vi "GSI-HVSwitch2.set high voltage.vi"(0 "i ref in":refnum<vi>, 2 "High Voltage":dbl format="%.2f", 3 "ms timeout (10000)":i32=10000, 5 "error in (no error)":errorcluster) -> (14 "i ref out":refnum<vi>, 17 "timed out":bool, 19 "error out":errorcluster)   [LabVIEW 2014, in "GSI-HVSwitch2.lvlib"]
doc: "Sets the voltage value for the logic \"High\" state."
uses:
  GSI-HVSwitch2.lvlib
  CSCore/CSSystem/CoreDefs/CoreDefs.error_type.ctl
  CSCore/CSSystem/CoreDefs/CoreDefs.error_severity.ctl
  CSlibraries-extern/DimLVEvent/LVDimInterface/LVDimInterface.lvlib
  CSCore/CSSystem/CoreLib/CoreLib.lvlib
  CSlibraries/UtilityLib/UtilityLib.lvlib
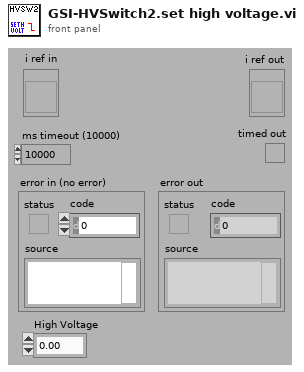
[diagram p1: front panel]
types:
  T1 = typedef "CoreDefs.error_severity.ctl" = enum16{"undefined", "information", "warning", "error", "fatal"}
  T2 = typedef "CoreDefs.error_type.ctl" = enum16{"no error", "can't load process", "can't unload process", "process does not exist", "can't install process", "can't remove process", "unknown function", "time out", "can't execute function", "duplicate queue name", "super not found", "caller queue invalid", "can't ping process", "unknown error", "VISA Error", "VISA timeout", "GPIB timeout", "GPIB error", "communication error", "data type mismatch", "can't read data from OPC server", "can't write data to OPC server", "OET error", "function not implemented", "process already exists", "invalid Shared Variable name", "error writing Shared Variable", "error reading Shared Variable", "invalid client name", "corrupt database", "unknown class", "call not authorized", "parameter out of range", "OET timeout: can't get data to modify", "invalid queue name", "requested operation incompatible with current state", "event undefined", "event disabled", "state undefined", "caller is not a friend", "EventBuilder: bad eventID", "EventBuilder: no DAQ devices", "a thread must not stop itself", "UNUSED ELEMENT4", "DiscArchiver: eventData incomplete", "DiscArchiver: eventData does not belong to run", "DiscArchiver: can't open file", "DiscArchiver: can't write to file", "DiscArchiver: available disc space low", "can't acquire semaphore", "error reading data from database", "notifier object is not existing", "can't register process", "can't unregister process", "illegal event type", "object disabled", "object already exists", "can't change state", "Instrument not found", "no connection to remote node", "invalid reference", "N/A", "UNUSED ELEMENT 1", "element not found", "illegal TCP/IP connection detected", "object does not exist", "invalid access ID", "unknown CS system", "invalid privilige", "unsupported data type", "unsupported server type", "IO server already exists", "Shared Variable already exists"}
  T3 = typedef "GSI-HVSwitch2.lvlib/GSI-HVSwitch2.i attribute.ctl" = cluster{"SDEX VISA Cluster":T4, "SetVoltage SW0":dbl, "SetVoltage SW1":dbl, "ActTempAmp":dbl, "ActTempPS1":dbl, "ActTempPS2":dbl, "mode":T7, "interfaceInitialized":bool, "serviceIDs":cluster{"nomVoltage0ID":i32, "nomVoltage1ID":i32, "actTempAmpID":i32, "actTempPS1ID":i32, "actTempPS2ID":i32, "modeID":i32}, "usedChannels":i32}
  T4 = typedef "SDEXDriver.lvlib/SDEX.VISA Control.ctl" = cluster{"VISA resource name":refnum<visa-resource-name>, "HEX address":u16, "VISA Timeout Value (1000 ms)":u32, "Lock Timeout (1000 ms)":u32, "semaphore":T5, "Baud rate":u32, "revision":T6, "deviceInfo":string}
  T5 = typedef "Semaphore RefNum" = refnum<k1>
  T6 = typedef "SDEXDriver.lvlib/SDEX.revisionType.ctl" = enum16{"unknown", "hvamp3", "hvswi1", "htrp0", "WDG0"}
  T7 = typedef "GSI-HVSwitch2.lvlib/GSI-HVSwitch2.mode.ctl" = enum16{"unknown", "switch", "stepper"}
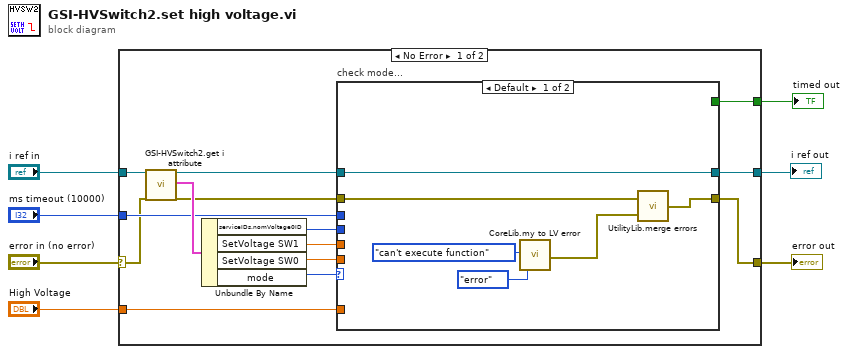
[diagram p0: block diagram]
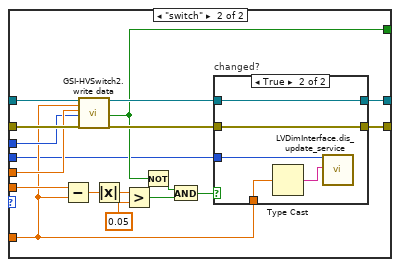
[diagram p2: hidden frame]
diagram:
  n1 = case shown="No Error" "error in (no error)" {
    selector: "error in (no error)" -> [w10 w53]
    tunnel: "i ref in" -> [w16 w54]
    tunnel: "ms timeout (10000)" -> [w15 _]
    tunnel: "High Voltage" -> [w14 _]
    tunnel: [w13 w54] -> w4
    tunnel: [w12 w53] -> w3
    tunnel: [w11 _] -> w2
    frame No Error {
      n2 = call "GSI-HVSwitch2.get i attribute.vi"("i ref in"=w16, "error in (no error)"=w10) -> ("i ref out"=w21:refnum<vi>, "i attribute"=w20:T3, "error out"=w19:errorcluster)  [unwired: 15 in]
      n3 = Unbundle By Name(w20) -> ("serviceIDs.nomVoltage0ID"=w9:i32, "SetVoltage SW1"=w18:dbl, "SetVoltage SW0"=w17:dbl, "mode"=w8:T7)
      n4 = case "check mode..." shown="Default" w8 {
        tunnel: w21 -> [w27 w45]
        tunnel: w19 -> [w24 w44]
        tunnel: w18 -> [_ w43]
        tunnel: w17 -> [_ w42]
        tunnel: w15 -> [_ w33]
        tunnel: w14 -> [_ w32]
        tunnel: [w27 w31] -> w13
        tunnel: [w22 w30] -> w12
        tunnel: [_ w29] -> w11
        tunnel: w9 -> [_ w28]
        frame Default {
          n5 = call "CoreLib.my to LV error.vi"("ErrorTypes"=CoreDefs.error_type."can't execute function", "severityLevel"=CoreDefs.error_severity."error") -> ("myErrorCluster"=w23:errorcluster)  [unwired: 16 in, 1 out]
          n6 = call "UtilityLib.merge errors.vi"("error2 (no error)"=w23, "error1 (no error)"=w24) -> ("error out"=w22:errorcluster)
        }
        frame "switch" {
          n7 = Subtract(x=w42, y=w32) -> (x-y=w41:dbl)
          n8 = call "GSI-HVSwitch2.write data.vi"("i ref in"=w45, "SetVoltage SW0"=w32, "SetVoltage SW1"=w43, "ms timeout (10000)"=w33, "error in (no error)"=w44) -> ("i ref out"=w36:refnum<vi>, "timed out"=w29:bool, "error out"=w37:errorcluster)  [unwired: 12 in]
          n9 = Absolute Value(x=w41) -> (abs(x)=w35:dbl)
          n10 = Greater?(x=w35, y=0.05) -> (0:w39:bool)
          n11 = Not(x=w29) -> (.not. x?=w40:bool)
          n12 = And(x=w40, y=w39) -> (x .and. y?=w38:bool)
          n13 = case "changed?" shown="True" w38 {
            tunnel: w37 -> [w47 w51]
            tunnel: [w47 w51] -> w30
            tunnel: w32 -> [_ w48]
            tunnel: w36 -> [w46 w52]
            tunnel: [w46 w52] -> w31
            tunnel: w28 -> [_ w50]
            frame False {
            }
            frame True {
              n14 = Type Cast(x=w48) -> (*(type *) &x=w49:string)  [unwired: 1 in]
              n15 = call "LVDimInterface.dis_update_service.vi"("my_serviceID"=w50, "data"=w49) -> ()  [unwired: 15 in, 3 out]
            }
          }
        }
      }
    }
    frame Error {
    }
  }
  "error out" <- w3
  "i ref out" <- w4
  "timed out" <- w2
